vi "Deserialize Core.vi"(8 "error in (no error)":errorcluster, 10 "Serialized Attributes":string, 11 "Serialize in":refnum<class "echo reply Msg.lvclass">) -> (0 "error out":errorcluster, 3 "Serialize out":refnum<class "echo reply Msg.lvclass">)   [LabVIEW 2020, in "Chat Window.lvlib" / "echo reply Msg.lvclass"]
uses:
  echo reply Msg.lvclass
  echo reply Msg.lvclass/echo reply Msg.ctl
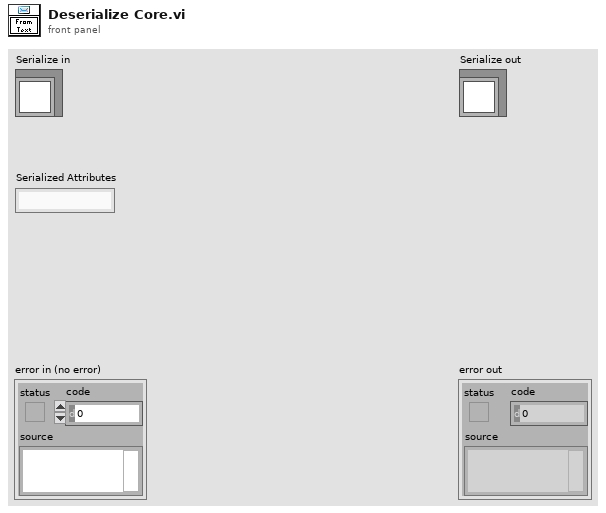
[diagram p1: front panel]
types:
  T1 = cluster{"Message":string, "id":string, "exec_time":i32}
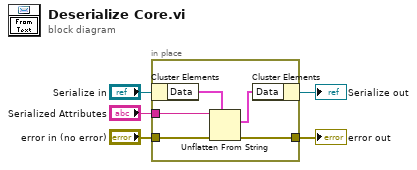
[diagram p0: block diagram]
diagram:
  n1 = in-place "In Place Element Structure" {
    in-place-border: "Serialized Attributes" -> [w6]
    in-place-border: "error in (no error)" -> [w8]
    in-place-border: [w7] -> w2
    n2 = in-place-cluster #1("Serialize in") -> ("Data"=w10:T1)
    n3 = Unflatten From String(type=w10, binary string=w6, error in (no error)=w8) -> (value=w9:T1, error out=w7:errorcluster)  [unwired: 2 in, 1 out]
    n4 = in-place-cluster #1("Data"=w9) -> (→"Serialize out":refnum<class "echo reply Msg.lvclass">)
  }
  "error out" <- w2
